vi "DAQ_SyncData.vi"(8 "Fehler (Eingang)":errorcluster, 11 "Data In":T1[](array[typedef])) -> (0 "Fehler (Ausgang)":errorcluster, 1 "Buffer length":i32, 2 "Data length":i32, 3 "Data Out":T1[](array[typedef]))   [LabVIEW 2016]
uses:
  DAQ_ReadBlock.ctl
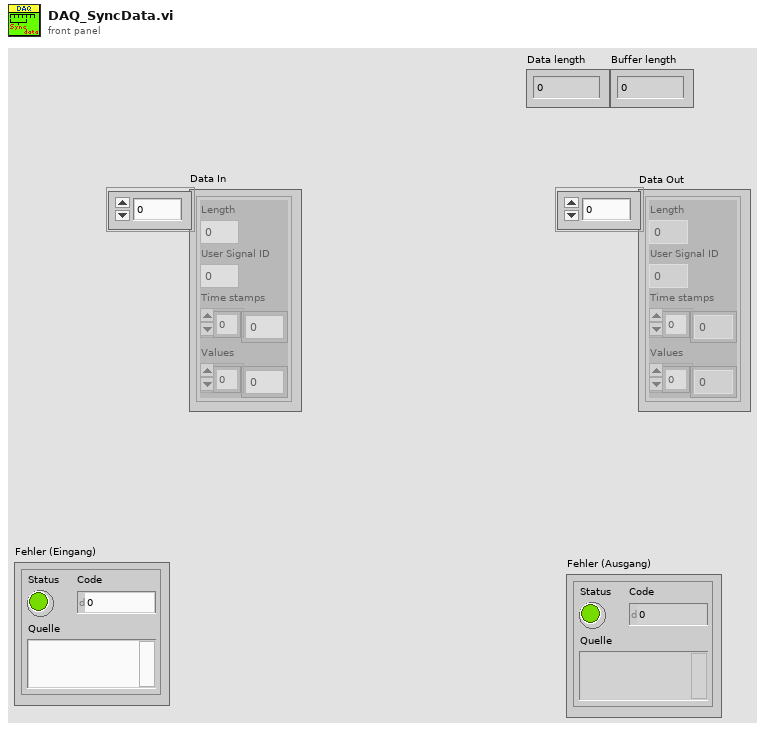
[diagram p1: front panel]
types:
  T1 = typedef "DAQ_ReadBlock.ctl" = cluster{"Length":i32, "User Signal ID":i32, "Time stamps":dbl[], "Values":dbl[]}
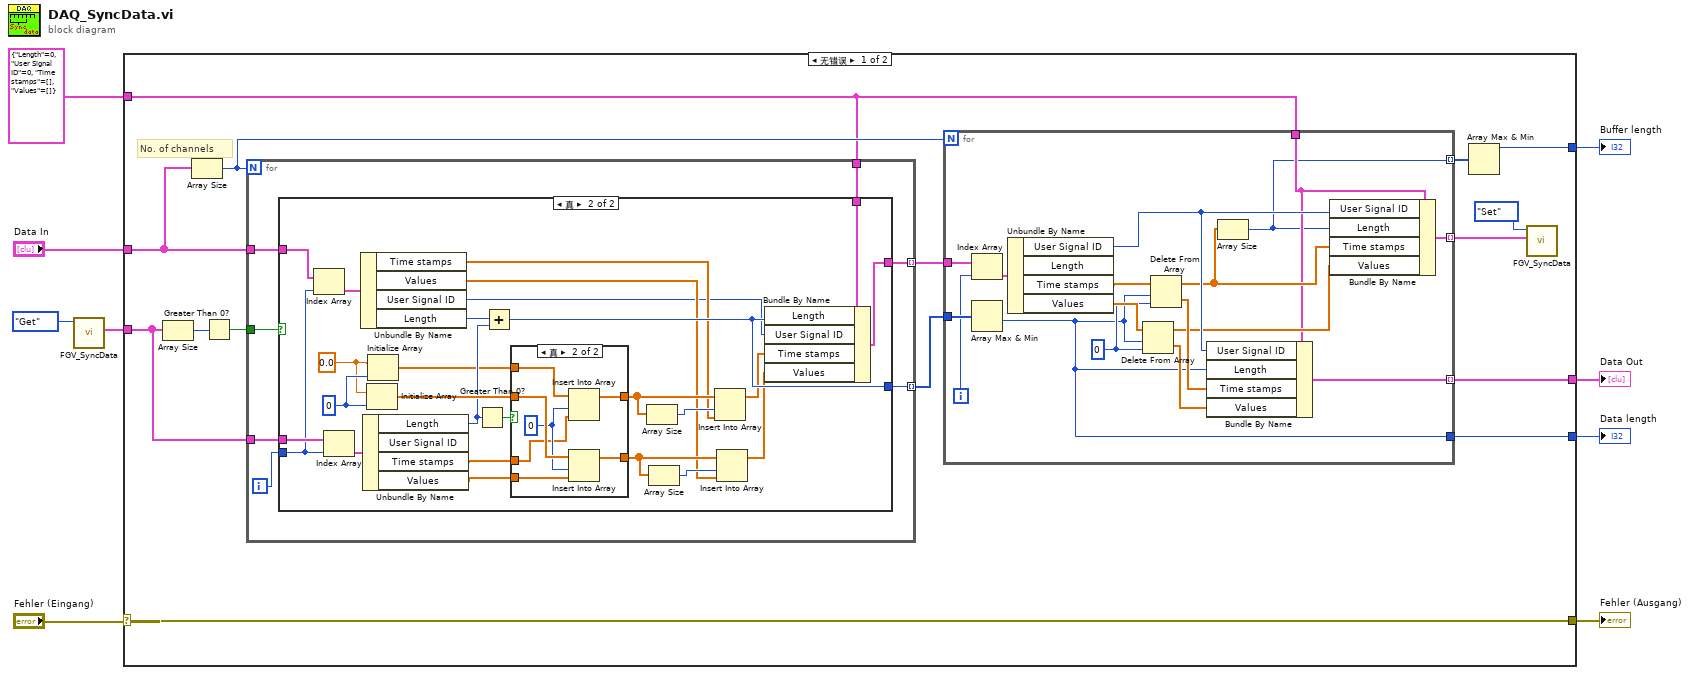
[diagram p0: block diagram]
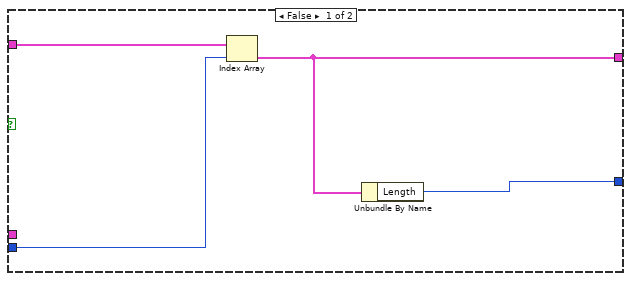
[diagram p2: hidden frame]
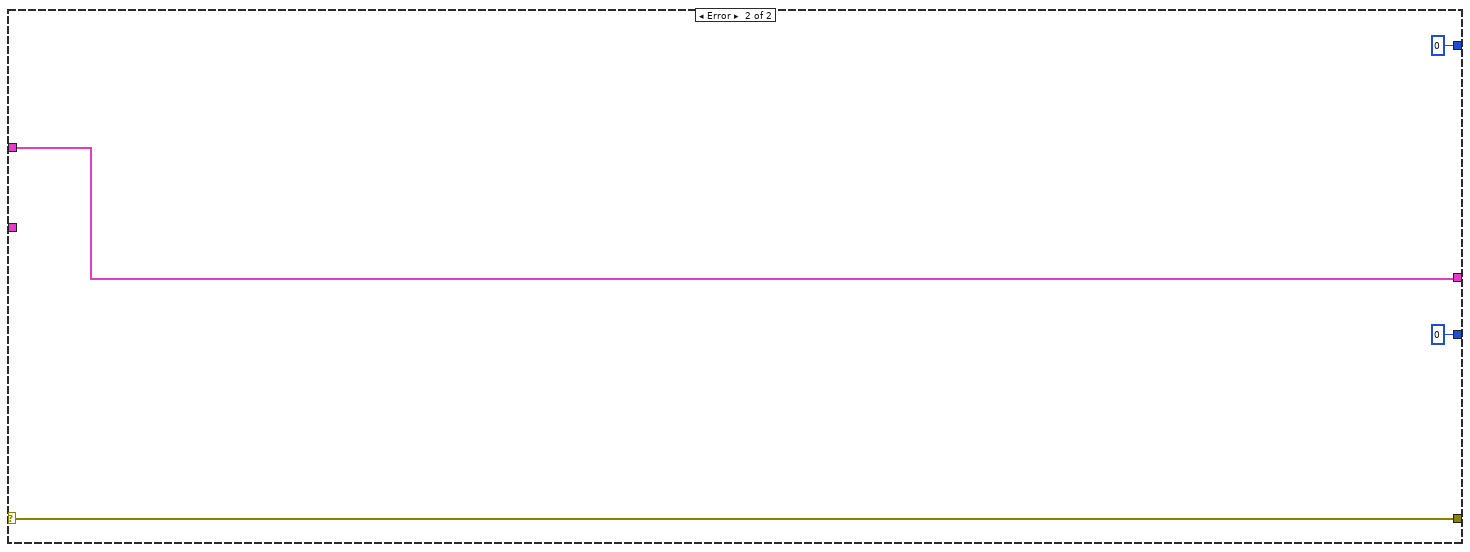
[diagram p4: hidden frame]
diagram:
  n1 = call "FGV_SyncData.vi"("Mode"=enum16{"Get", "Set", "Init"}."Get") -> ("Data out"=w6:T1[])  [unwired: 10 in]
  n2 = case shown="无错误" "Fehler (Eingang)" {
    selector: "Fehler (Eingang)" -> [w24 w91]
    tunnel: [w24 w91] -> w8
    tunnel: "Data In" -> [w20 w90]
    tunnel: w6 -> [w21 _]
    tunnel: [w15 w90] -> w5
    tunnel: T1 {"Length"=0, "User Signal ID"=0, "Time stamps"=[], "Values"=[]} ("Read block") -> [w13 _]
    tunnel: [w12 0] -> w2
    tunnel: [w10 0] -> w1
    frame No Error {
      # "No. of channels"
      n3 = Array Size(array=w21) -> (size(s)=w23:i32)
      n4 = Array Size(array=w20) -> (size(s)=w19:i32)
      n5 = Greater Than 0?(x=w23) -> (x > 0?=w22:bool)
      n6 = for {
        N: w19 -> [_]
        tunnel: w20 -> [w47]
        tunnel: w22 -> [w48]
        tunnel: w21 -> [w46]
        tunnel: [w45] -> w18 mode=indexing
        tunnel: [w43] -> w17 mode=indexing
        tunnel: w13 -> [w42]
        i -> [w44]
        n7 = case shown="真" w48 {
          tunnel: w47 -> [w52 w78]
          tunnel: w44 -> [w51 w75]
          tunnel: [w50 w67] -> w45
          tunnel: w46 -> [_ w76]
          tunnel: [w49 w66] -> w43
          tunnel: w42 -> [_ w53]
          frame False {
            n8 = Index Array(array=w52, index=w51) -> (element=w50:T1)
            n9 = Unbundle By Name(w50) -> ("Length"=w49:i32)
          }
          frame True {
            w64 = 0.0
            w65 = 0 ("Dimension")
            n10 = Index Array(array=w78, index=w75) -> (element=w77:T1)
            n11 = Index Array(array=w76, index=w75) -> (element=w74:T1)
            n12 = Unbundle By Name(w77) -> ("Time stamps"=w58:dbl[], "Values"=w57:dbl[], "User Signal ID"=w54:i32, "Length"=w68:i32)
            n13 = Unbundle By Name(w74) -> ("Length"=w69:i32, "Time stamps"=w62:dbl[], "Values"=w61:dbl[])  [unwired: 1 out]
            n14 = Initialize Array(w64, w65) -> (w72:dbl[])
            n15 = Initialize Array(w64, w65) -> (w63:dbl[])
            n16 = Greater Than 0?(x=w69) -> (x > 0?=w73:bool)
            n17 = Add(x=w68, y=w69) -> (x+y=w66:i32)
            n18 = case shown="真" w73 {
              tunnel: w72 -> [w79 w85]
              tunnel: [w80 w86] -> w70
              tunnel: w63 -> [w80 w87]
              tunnel: w62 -> [_ w82]
              tunnel: w61 -> [_ w83]
              tunnel: [w79 w81] -> w59
              frame False {
              }
              frame True {
                w84 = 0 ("Index")
                n19 = Insert Into Array(array=w87, index=w84, new element=w82) -> (w86:dbl[])
                n20 = Insert Into Array(array=w85, index=w84, new element=w83) -> (w81:dbl[])
              }
            }
            n21 = Array Size(array=w70) -> (size(s)=w71:i32)
            n22 = Array Size(array=w59) -> (size(s)=w60:i32)
            n23 = Insert Into Array(array=w70, index=w71, new element=w58) -> (w56:dbl[])
            n24 = Insert Into Array(array=w59, index=w60, new element=w57) -> (w55:dbl[])
            n25 = Bundle By Name(cluster=w53, "Length"=w66, "User Signal ID"=w54, "Time stamps"=w56, "Values"=w55) -> (w67:T1)
          }
        }
      }
      n26 = for {
        N: w19 -> [_]
        tunnel: w18 -> [w40]
        tunnel: w17 -> [w39]
        tunnel: [w36] -> w16 mode=indexing
        tunnel: [w35] -> w15 mode=indexing
        tunnel: w13 -> [w27]
        tunnel: [w26] -> w12
        tunnel: [w25] -> w11 mode=indexing
        i -> [w34]
        w30 = 0 ("Index")
        n27 = Index Array(array=w40, index=w34) -> (element=w41:T1)
        n28 = Array Max & Min(array=w39) -> (min value=w26:i32)  [unwired: 3 out]
        n29 = Unbundle By Name(w41) -> ("User Signal ID"=w38:i32, "Time stamps"=w33:dbl[], "Values"=w31:dbl[])  [unwired: 1 out]
        n30 = Delete From Array(array=w31, length=w26, index=w30) -> (deleted portion=w29:dbl[], array with subset deleted=w28:dbl[])
        n31 = Delete From Array(array=w33, length=w26, index=w30) -> (deleted portion=w32:dbl[], array with subset deleted=w37:dbl[])
        n32 = Bundle By Name(cluster=w27, "User Signal ID"=w38, "Length"=w26, "Time stamps"=w32, "Values"=w29) -> (w35:T1)
        n33 = Array Size(array=w37) -> (size(s)=w25:i32)
        n34 = Bundle By Name(cluster=w27, "User Signal ID"=w38, "Length"=w25, "Time stamps"=w37, "Values"=w28) -> (w36:T1)
      }
      n35 = Array Max & Min(array=w11) -> (max value=w10:i32)  [unwired: 3 out]
      n36 = call "FGV_SyncData.vi"("Data In"=w16, "Mode"=enum16{"Get", "Set", "Init"}."Set") -> ()  [unwired: 9 in, 1 out]
    }
    frame Error {
    }
  }
  "Fehler (Ausgang)" <- w8
  "Data Out" <- w5
  "Data length" <- w2
  "Buffer length" <- w1
